vi "E7_20_write.vi"(6 "Command":T6, 8 "error in":T7, 11 "DriverConnect in":T1={"InterfaceType"=enum."VISA", "OpenedSession"="", "InterfaceSettings"={"Interface"=enum."RS232", "EOS 4 read"=enum."LF (\\n)", "EOS 4 write"=enum."LF (\\n)", "TMO, ms"=10000, "Sett"=variant(cluster{"Baud Rate":u32, "Data Bits":u16, "Parity":u16, "Stop Bits":u16, "Flow Control":u16, "Eho":bool} {"Baud Rate"=75, "Data Bits"=0, "Parity"=0, "Stop Bits"=0, "Flow Control"=0, "Eho"=FALSE})}}) -> (0 "error out":T7, 3 "DriverConnect out":T1={"InterfaceType"=enum."VISA", "OpenedSession"="", "InterfaceSettings"={"Interface"=enum."RS232", "EOS 4 read"=enum."LF (\\n)", "EOS 4 write"=enum."LF (\\n)", "TMO, ms"=10000, "Sett"=variant(cluster{"Baud Rate":u32, "Data Bits":u16, "Parity":u16, "Stop Bits":u16, "Flow Control":u16, "Eho":bool} {"Baud Rate"=75, "Data Bits"=0, "Parity"=0, "Stop Bits"=0, "Flow Control"=0, "Eho"=FALSE})}})   [LabVIEW 2018]
uses:
  MOKO_LabViewLibrary/MokoLowLevel/MokoLowLovelControl/MLLC_Error.ctl
  MOKO_LabViewLibrary/MokoLowLevel/MokoLowLovelControl/MLLC_Command.ctl
  MOKO_LabViewLibrary/MokoLowLevel/MokoLowLovelControl/MLLC_ConnectCluster.ctl
  MOKO_LabViewLibrary/MokoLowLevel/MokoLowLovelControl/MLLC_InterfaceType.ctl
  MOKO_LabViewLibrary/MokoLowLevel/MokoLowLovelControl/MLLC_OpenedSession.ctl
  MOKO_LabViewLibrary/MokoLowLevel/MokoLowLovelControl/MLLC_InterfaceSettings.ctl
  MOKO_LabViewLibrary/MokoLowLevel/MokoLowLovelControl/MLLC_InterfaceKind.ctl
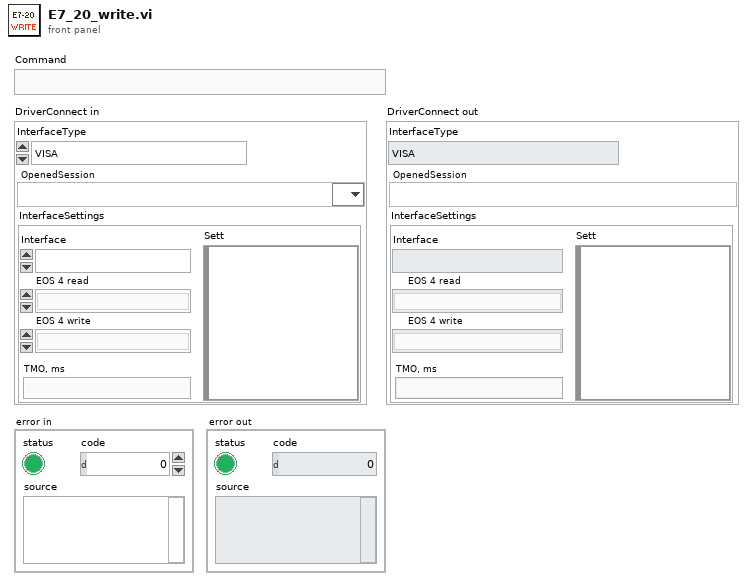
[diagram p1: front panel]
types:
  T1 = typedef "MLLC_ConnectCluster.ctl" = cluster{"InterfaceType":T2, "OpenedSession":T3, "InterfaceSettings":T4}
  T2 = typedef "MLLC_InterfaceType.ctl" = enum16{"VISA", "Prologix USB-GPIB"}
  T3 = typedef "MLLC_OpenedSession.ctl" = refnum<visa-resource-name>
  T4 = typedef "MLLC_InterfaceSettings.ctl" = cluster{"Interface":T5, "EOS 4 read":enum16{"Default (=EOS 4 write)", "CR (\\r)", "LF (\\n)", "None"}, "EOS 4 write":enum16{"CR+LF (\\r\\n)", "CR (\\r)", "LF (\\n)", "None"}, "TMO, ms":i32, "Sett":variant}
  T5 = typedef "MLLC_InterfaceKind.ctl" = enum16{"RS232", "GPIB", "USB", "Ethernet", "another"}
  T6 = typedef "MLLC_Command.ctl" = string
  T7 = typedef "MLLC_Error.ctl" = errorcluster
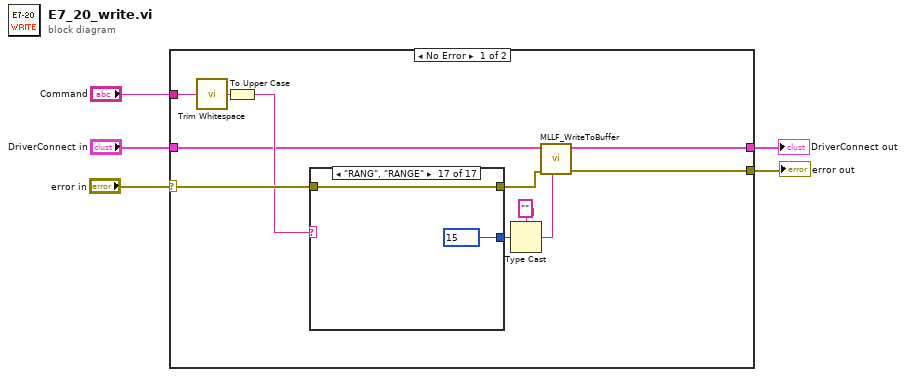
[diagram p0: block diagram]
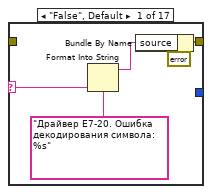
[diagram p2: hidden frame]
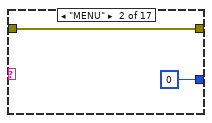
[diagram p3: hidden frame]
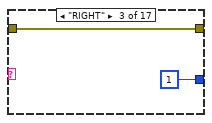
[diagram p4: hidden frame]
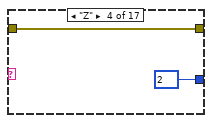
[diagram p5: hidden frame]
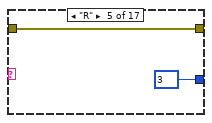
[diagram p6: hidden frame]
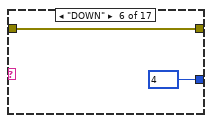
[diagram p7: hidden frame]
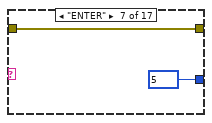
[diagram p8: hidden frame]
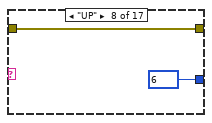
[diagram p9: hidden frame]
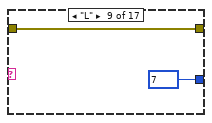
[diagram p10: hidden frame]
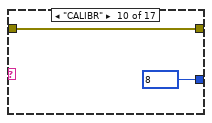
[diagram p11: hidden frame]
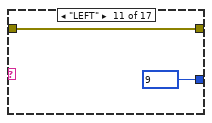
[diagram p12: hidden frame]
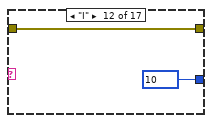
[diagram p13: hidden frame]
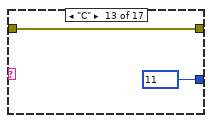
[diagram p14: hidden frame]
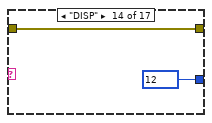
[diagram p15: hidden frame]
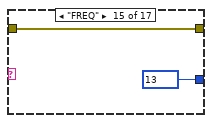
[diagram p16: hidden frame]
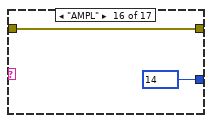
[diagram p17: hidden frame]
diagram:
  n1 = case shown="No Error" "error in" {
    selector: "error in" -> [w16 w55]
    tunnel: [w10 w55] -> w5
    tunnel: [w11 w54] -> w1
    tunnel: "Command" -> [w8 _]
    tunnel: "DriverConnect in" -> [w6 w54]
    frame No Error {
      n2 = call <vilib>:"Trim Whitespace.vi"("string"=w8) -> ("trimmed string"=w9:string)  [unwired: 1 in]
      n3 = To Upper Case(1:w9) -> (0:w7:string)
      n4 = case shown="\"RANG\", \"RANGE\"" w7 {
        selector: w7 -> [w18 _ _ _ _ _ _ _ _ _ _ _ _ _ _ _ _]
        tunnel: [w20 w23 w25 w27 w29 w31 w33 w35 w37 w39 w41 w43 w45 w47 w49 w51 w53] -> w15
        tunnel: w16 -> [_ w23 w25 w27 w29 w31 w33 w35 w37 w39 w41 w43 w45 w47 w49 w51 w53]
        tunnel: [_ u8 0 ("length (rest)") u8 1 ("length (rest)") u8 2 ("length (rest)") u8 3 ("length (rest)") u8 4 ("length (rest)") u8 5 ("length (rest)") u8 6 ("length (rest)") u8 7 ("length (rest)") u8 8 ("length (rest)") u8 9 ("length (rest)") u8 10 ("length (rest)") u8 11 ("length (rest)") u8 12 ("length (rest)") u8 13 ("length (rest)") u8 14 ("length (rest)") u8 15 ("length (rest)")] -> w12
        frame "False", Default {
          n5 = Format Into String(format string="Драйвер Е7-20. Ошибка декодирования символа: %s" ("source"), w18) -> (resulting string=w19:string)  [unwired: 2 in, 1 out]
          n6 = Bundle By Name(cluster=errorcluster {"status"=TRUE, "code"=5436, "source"="Драйвер Г5-82. Ошибка декодирования символа: %s"} ("error IO"), "source"=w19) -> (w20:errorcluster)
        }
        frame "MENU" {
        }
        frame "RIGHT" {
        }
        frame "Z" {
        }
        frame "R" {
        }
        frame "DOWN" {
        }
        frame "ENTER" {
        }
        frame "UP" {
        }
        frame "L" {
        }
        frame "CALIBR" {
        }
        frame "LEFT" {
        }
        frame "I" {
        }
        frame "C" {
        }
        frame "DISP" {
        }
        frame "FREQ" {
        }
        frame "AMPL" {
        }
        frame "RANG", "RANGE" {
        }
      }
      n7 = Type Cast(type="", x=w12) -> (*(type *) &x=w14:string)
      n8 = call "MLLF_WriteToBuffer.vi"("String"=w14, "error in"=w15, "DriverConnect in"=w6) -> ("error out"=w10:T7, "DriverConnect out"=w11:T1)  [unwired: 5 in]
    }
    frame Error {
    }
  }
  "error out" <- w5
  "DriverConnect out" <- w1
